vi "Usb_Relay_Gpio_LV24.vi"() -> ()   [LabVIEW 2024]
uses:
  <vilib>/Instr/_visa.llb/VISA Configure Serial Port (Instr).vi
panel:
  out "Instruction 3":string="3. Result will be displaed below."
  out "Instruction 2":string="2. Press the run button on the Frontpanel"
  out "Instruction 1":string="1. Please enter the COM Port and the command to execute." caption="String"
  in  "Command":string
  out "Output":string
  in  "COM Port":refnum<visa-resource-name>
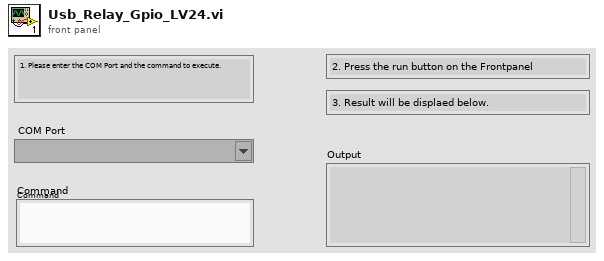
[diagram p1: front panel]
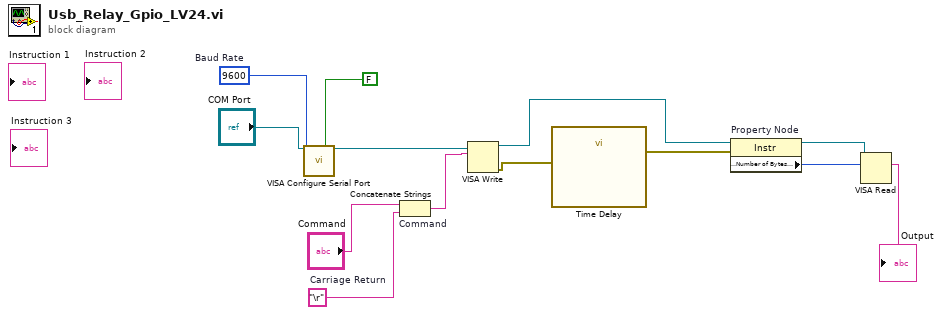
[diagram p0: block diagram]
diagram:
  w1 = u32 9600  # Baud Rate
  w3 = "\r"  # Carriage Return
  n1 = call-poly "VISA Configure Serial Port"("VISA resource name"="COM Port", "Enable Termination\nChar (T)"=FALSE ("Enable Termination\nChar (T)"), "baud rate (9600)"=w1) -> ("VISA resource name out"=w2:refnum<visa-resource-name>)  [unwired: 11 in, 1 out]
  n2 = Concatenate Strings "Command"("Command", w3) -> (w5:string)
  n3 = VISA Write(VISA resource name=w2, write buffer=w5) -> (VISA resource name out=w6:refnum<visa-resource-name>, error out=w8:errorcluster)  [unwired: 1 in, 1 out]
  n4 = call "Time Delay"("error in (no error)"=w8) -> ("error out"=w7:errorcluster)  [unwired: 10 in]
  n5 = property on="Property Node" class="Instr"(reference=w6, error in=w7) -> (reference out=w11:refnum<visa-resource-name>, "Serial Settings:Number of Bytes at Serial Port"=w10:u32)  [unwired: 1 out]
  n6 = VISA Read(VISA resource name=w11, byte count=w10) -> (read buffer=→"Output":string)  [unwired: 1 in, 3 out]
